vi "Remove Device from Stack.vi"(7 "Device":refnum<class "Device.lvclass">, 8 "error in (no error)":errorcluster, 11 "Stack in":refnum<class "Device.lvclass">[](array[class])) -> (0 "error out":errorcluster, 3 "Stack out":refnum<class "Device.lvclass">[](array[class]))   [LabVIEW 2011, in "Tinkerforge.lvlib" / "Device.lvclass"]
doc: "This VI updates the stack and removes the <B>Device</B> from the <B>Stack</B>."
uses:
  Device.lvclass
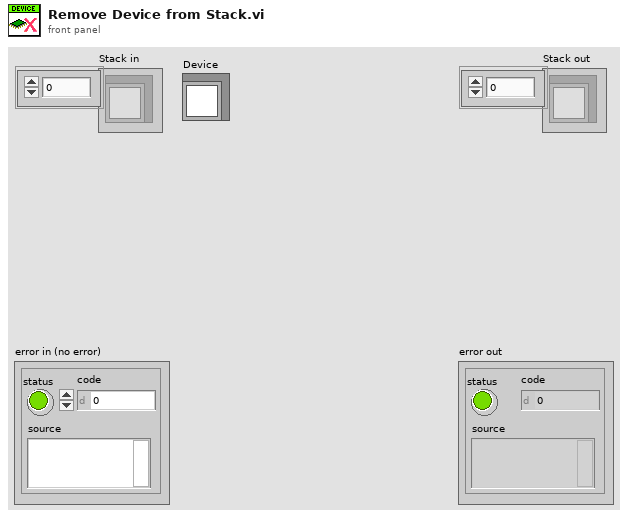
[diagram p1: front panel]
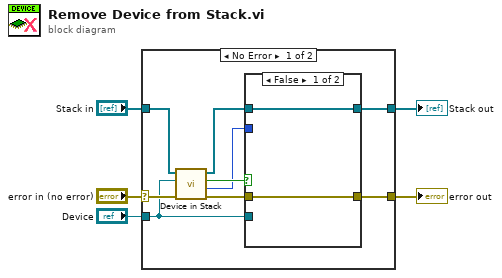
[diagram p0: block diagram]
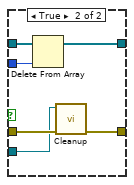
[diagram p2: hidden frame]
diagram:
  n1 = case shown="No Error" "error in (no error)" {
    selector: "error in (no error)" -> [w14 w24]
    tunnel: [w6 w24] -> w4
    tunnel: [w9 w23] -> w2
    tunnel: "Stack in" -> [w12 w23]
    tunnel: "Device" -> [w7 _]
    frame No Error {
      n2 = call "Device in Stack.vi"("error in (no error)"=w14, "Device in"=w7, "Stack in"=w12) -> ("error out"=w8:errorcluster, "Stack Index"=w10:i32, "Device found?"=w13:bool, "Stack out"=w11:refnum<class "Device.lvclass">[])  [unwired: 5 in]
      n3 = case shown="False" w13 {
        tunnel: w11 -> [w16 w22]
        tunnel: w10 -> [_ w21]
        tunnel: [w16 w20] -> w9
        tunnel: w8 -> [w15 w19]
        tunnel: w7 -> [_ w18]
        tunnel: [w15 w17] -> w6
        frame False {
        }
        frame True {
          n4 = Delete From Array(array=w22, index=w21) -> (array with subset deleted=w20:refnum<class "Device.lvclass">[])  [unwired: 1 in, 1 out]
          n5 = call-dynamic "Cleanup.vi"("error in (no error)"=w19, "Device in"=w18) -> ("error out"=w17:errorcluster)  [unwired: 9 in]
        }
      }
    }
    frame Error {
    }
  }
  "error out" <- w4
  "Stack out" <- w2
